vi "PPFS_DRIVE_ORIENT_CORRECT.vi"(9 "FPGA_Time_Seconds":dbl, 10 "Gyro Heading Radians":dbl, 11 "Drv Rotation Orentation Dmd  Radians":dbl) -> (3 "CO-ControlOutput":dbl)   [LabVIEW 2019]
uses:
  <vilib>/Rock Robotics/WPI/ThirdParty/JAS_Junk/TrajLib/TypeDef/X_Y_PAIR.ctl
  <vilib>/Rock Robotics/WPI/ThirdParty/JAS_Junk/TrajLib/MathUtil_InputModulus.vi
  <vilib>/Rock Robotics/WPI/ThirdParty/JAS_Junk/TrajLib/VI/Util_GetTime_U32.vi
  <vilib>/Rock Robotics/WPI/ThirdParty/JAS_Junk/TrajLib/VI/FunctionGenerator_New.vi
  <vilib>/Rock Robotics/WPI/ThirdParty/JAS_Junk/TrajLib/VI/FunctionGenerator_Calculate.vi
  <vilib>/Rock Robotics/WPI/ThirdParty/JAS_Junk/TrajLib/PIDController_AtSetpoint.vi
  <vilib>/Rock Robotics/WPI/ThirdParty/JAS_Junk/TrajLib/PIDController_SetPIDF.vi
  <vilib>/Rock Robotics/WPI/ThirdParty/JAS_Junk/TrajLib/PIDController_SetDerivativeFilter.vi
  <vilib>/Rock Robotics/WPI/ThirdParty/JAS_Junk/TrajLib/PIDController_SetIntegratorRange.vi
  <vilib>/Rock Robotics/WPI/ThirdParty/JAS_Junk/TrajLib/PIDController_SetTolerancePandV.vi
  <vilib>/Rock Robotics/WPI/ThirdParty/JAS_Junk/TrajLib/PIDController_DisableContinousInput.vi
  <vilib>/Rock Robotics/WPI/ThirdParty/JAS_Junk/TrajLib/PIDController_EnableContinousInput.vi
  <vilib>/Rock Robotics/WPI/ThirdParty/JAS_Junk/TrajLib/PIDController_Reset.vi
  <vilib>/Rock Robotics/WPI/ThirdParty/JAS_Junk/TrajLib/PIDController_New.vi
  <vilib>/Rock Robotics/WPI/ThirdParty/JAS_Junk/TrajLib/PIDController_SetOutputLimits.vi
  <vilib>/Rock Robotics/WPI/ThirdParty/JAS_Junk/TrajLib/VI/PIDController_SetIntegratorZone.vi
  <vilib>/Rock Robotics/WPI/ThirdParty/JAS_Junk/TrajLib/PIDController_NewPeriod.vi
  <vilib>/Rock Robotics/SystemInterfaces/NetworkCommunication/NetComm_UsageReport_report.vi
  <vilib>/Rock Robotics/WPI/ThirdParty/JAS_Junk/TrajLib/VI/Util_GetTime_U64.vi
  PPFS_DRIVE_GLOBALS.vi
  <vilib>/gmath/interp.llb/Search Ordered Table.vi
  <vilib>/Rock Robotics/WPI/ThirdParty/JAS_Junk/TrajLib/Globals/Util_LibraryGlobals.vi
  <vilib>/Rock Robotics/WPI/ThirdParty/JAS_Junk/TrajLib/PIDController_AdvCalculate_FF_Sp_Pv.vi
  <vilib>/Rock Robotics/WPI/ThirdParty/JAS_Junk/TrajLib/Trajectory_Library.lvlib
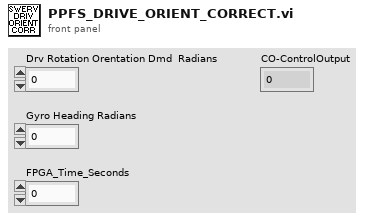
[diagram p1: front panel]
types:
  T1 = typedef "Trajectory_Library.lvlib/X_Y_PAIR.ctl" = cluster{"X":dbl, "Y":dbl}
  T2 = typedef "Trajectory_Library.lvlib/PID_ADV_LIMITS.ctl" = cluster{"MaxInput":dbl, "MinInput":dbl, "Continuous":bool, "MaxOutput":dbl, "MinOutput":dbl}
  T3 = typedef "Trajectory_Library.lvlib/PID_ADV_TUNING.ctl" = cluster{"Kf":dbl, "Kp":dbl, "Ki":dbl, "Kd":dbl, "MaximumIntegral":dbl, "MinimumIntegral":dbl, "Filter Derivative":bool, "IntegralZone":dbl}
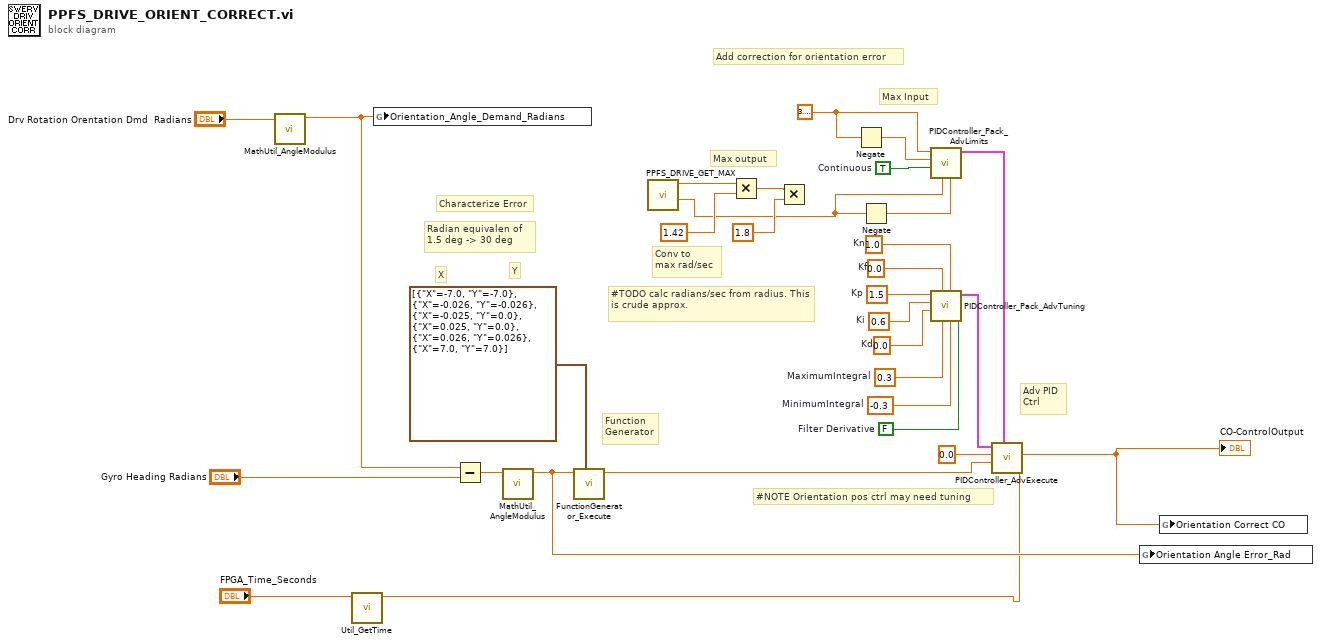
[diagram p0: block diagram]
diagram:
  w18 = 3.141592653589793
  w7 = 1.0  # Kn
  w8 = 1.5  # Kp
  w9 = 0.6  # Ki
  w10 = 0.0  # Kd
  w11 = 0.0  # Kf
  w12 = 0.3  # MaximumIntegral
  w13 = -0.3  # MinimumIntegral
  w14 = FALSE  # Filter Derivative
  w15 = TRUE  # Continuous
  # "Add correction for orientation error"
  # "Characterize Error"
  # "Conv to\nmax rad/sec"
  # "Max output"
  # "Max Input"
  # "Adv PID\nCtrl"
  # "Radian equivalen of \n1.5 deg -> 30 deg"
  # "Function\nGenerator"
  # "Y"
  # "X"
  # "#TODO calc radians/sec from radius. This is crude approx."
  # "#NOTE Orientation pos ctrl may need tuning"
  n1 = call <vilib>:"MathUtil_AngleModulus.vi"("InputAngle"="Drv Rotation Orentation Dmd  Radians") -> ("ModulsAngle"=w4:dbl)  [unwired: 10 in]
  n2 = call <vilib>:"Util_GetTime.vi"("Pass_Through_Time"="FPGA_Time_Seconds") -> ("FPGA_Time_Seconds"=w2:dbl)  [unwired: 8 in, 2 out]
  n3 = global write "PPFS_DRIVE_GLOBALS.vi" "Orientation_Angle_Demand_Radians"(w4) -> ()
  n4 = Subtract(x=w4, y="Gyro Heading Radians") -> (x-y=w27:dbl)
  n5 = call <vilib>:"MathUtil_AngleModulus.vi"("InputAngle"=w27) -> ("ModulsAngle"=w29:dbl)  [unwired: 10 in]
  n6 = call <vilib>:"FunctionGenerator_Execute.vi"("X Y Pairs"=T1[] [{"X"=-7.0, "Y"=-7.0}, {"X"=-0.026, "Y"=-0.026}, {"X"=-0.025, "Y"=0.0}, {"X"=0.025, "Y"=0.0}, {"X"=0.026, "Y"=0.026}, {"X"=7.0, "Y"=7.0}], "Input Value"=w29) -> ("Output Value"=w28:dbl)  [unwired: 9 in]
  n7 = call "PPFS_DRIVE_GET_MAX.vi"() -> ("Max Rotational Vel (Rad/Sec)"=w1:dbl, "Max Wheel Vel (Meter/Sec)"=w21:dbl)  [unwired: 10 in]
  n8 = Multiply(x=w21, y=1.42) -> (x*y=w22:dbl)
  n9 = Multiply(x=w22, y=1.8) -> ()  [unwired: 1 out]
  n10 = Negate(x=w18) -> (-x=w19:dbl)
  n11 = Negate(x=w1) -> (-x=w24:dbl)
  n12 = call <vilib>:"PIDController_Pack_AdvLimits.vi"("MinOutput"=w24, "MaxOutput"=w1, "Continuous"=w15, "MinInput"=w19, "MaxInput"=w18) -> ("Adv PID Limits"=w17:T2)  [unwired: 6 in]
  n13 = call <vilib>:"PIDController_Pack_AdvTuning.vi"("Filter Derivative"=w14, "MinimumIntegral"=w13, "Kn"=w7, "MaximumIntegral"=w12, "Kf"=w11, "Kd"=w10, "Ki"=w9, "Kp"=w8) -> ("Adv PID Tuning"=w16:T3)  [unwired: 3 in]
  n14 = call <vilib>:"PIDController_AdvExecute.vi"("Time"=w2, "Adv PID Limits"=w17, "SP-SetPoint"=w28, "PV-Measurement"=0.0, "Adv PID Tuning"=w16) -> ("CO-ControlOutput"=w26:dbl)  [unwired: 4 in, 2 out]
  "CO-ControlOutput" <- w26
  n15 = global write "PPFS_DRIVE_GLOBALS.vi" "Orientation Angle Error_Rad"(w29) -> ()
  n16 = global write "PPFS_DRIVE_GLOBALS.vi" "Orientation Correct CO"(w26) -> ()
